vi "Measurements Graph_Seperated Ports.vi"(0 "Resitance":dbl[](array[numeric])=[0.1, 0.1, 0.3, 0.28, 0.18, 0.08], 1 "Bias Voltage":dbl[](array[numeric])=[0.0, 1.0, 2.0, 2.0, 1.0, 0.0], 2 "Stop_V":dbl, 5 "P1":dbl[](array[numeric])=[10.0, 11.0, 12.0, 11.75, 10.85, 9.5], 7 "P2":dbl[](array[numeric])=[20.0, 21.0, 22.0, 21.75, 20.35, 18.65], 9 "P3":dbl[](array[numeric])=[30.0, 31.0, 32.0, 31.5, 30.47, 29.42], 11 "Error In":errorcluster) -> (4 "Graph Cluster":T1, 15 "Error Out":errorcluster)   [LabVIEW 2013]
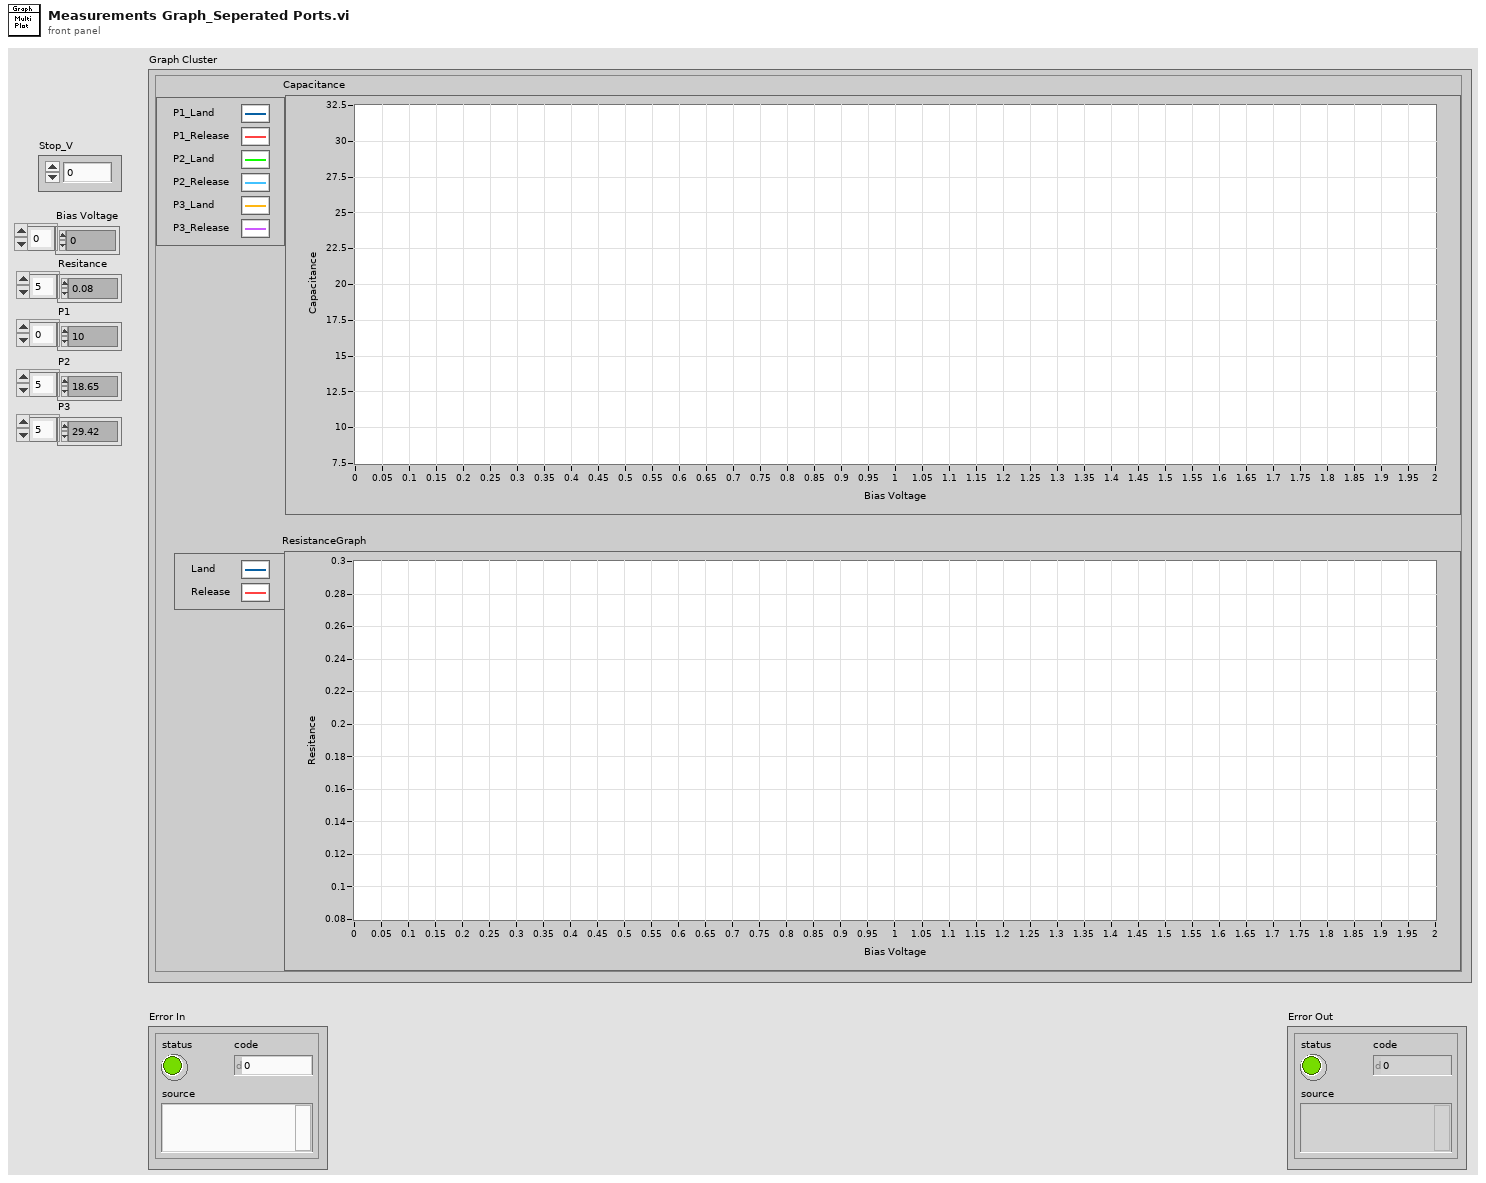
[diagram p1: front panel]
types:
  T1 = cluster{"ResistanceGraph":cluster{dbl[], dbl[]}[], "Capacitance":cluster{dbl[], dbl[]}[]}
  T2 = cluster{cluster{dbl[], dbl[]}[], cluster{dbl[], dbl[]}[]}
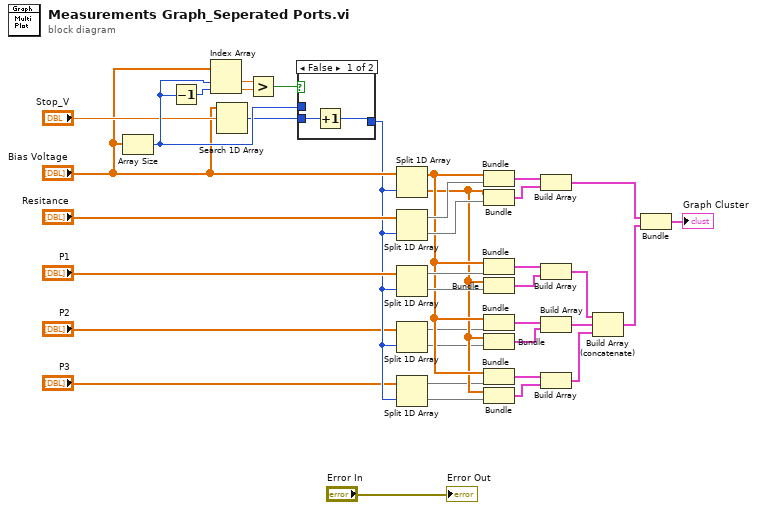
[diagram p0: block diagram]
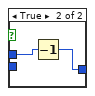
[diagram p2: hidden frame]
diagram:
  n1 = Array Size(array="Bias Voltage") -> (size(s)=w24:i32)
  n2 = Decrement(x=w24) -> (x-1=w27:i32)
  n3 = Index Array(array="Bias Voltage", index #1=w24, index #2=w27) -> (element #1=w25:dbl, element #2=w26:dbl)
  n4 = Search 1D Array(1D array="Bias Voltage", element="Stop_V") -> (index of element=w21:i32)  [unwired: 1 in]
  n5 = Greater?(x=w25, y=w26) -> (0:w20:bool)
  n6 = case shown="False" w20 {
    tunnel: w24 -> [_ w42]
    tunnel: [w39 w41] -> w17
    tunnel: w21 -> [w40 _]
    frame False {
      n7 = Increment(x=w40) -> (x+1=w39:i32)
    }
    frame True {
      n8 = Decrement(x=w42) -> (x-1=w41:i32)
    }
  }
  n9 = Split 1D Array(array="Bias Voltage", index=w17) -> (first subarray=w15:dbl[], second subarray=w14:dbl[])
  n10 = Split 1D Array(array="Resitance", index=w17) -> (first subarray=w37:dbl[], second subarray=w36:dbl[])
  n11 = Split 1D Array(array="P1", index=w17) -> (first subarray=w31:dbl[], second subarray=w30:dbl[])
  n12 = Split 1D Array(array="P2", index=w17) -> (first subarray=w13:dbl[], second subarray=w12:dbl[])
  n13 = Split 1D Array(array="P3", index=w17) -> (first subarray=w11:dbl[], second subarray=w10:dbl[])
  n14 = Bundle(w15, w37) -> (w35:cluster{dbl[], dbl[]})  [unwired: 1 in]
  n15 = Bundle(w14, w36) -> (w34:cluster{dbl[], dbl[]})  [unwired: 1 in]
  n16 = Bundle(w15, w31) -> (w33:cluster{dbl[], dbl[]})  [unwired: 1 in]
  n17 = Bundle(w14, w30) -> (w32:cluster{dbl[], dbl[]})  [unwired: 1 in]
  n18 = Bundle(w15, w13) -> (w8:cluster{dbl[], dbl[]})  [unwired: 1 in]
  n19 = Bundle(w14, w12) -> (w7:cluster{dbl[], dbl[]})  [unwired: 1 in]
  n20 = Bundle(w15, w11) -> (w6:cluster{dbl[], dbl[]})  [unwired: 1 in]
  n21 = Bundle(w14, w10) -> (w5:cluster{dbl[], dbl[]})  [unwired: 1 in]
  n22 = Build Array(w35, w34) -> (w29:cluster{dbl[], dbl[]}[])
  n23 = Build Array(w33, w32) -> (w4:cluster{dbl[], dbl[]}[])
  n24 = Build Array(w8, w7) -> (w3:cluster{dbl[], dbl[]}[])
  n25 = Build Array(w6, w5) -> (w2:cluster{dbl[], dbl[]}[])
  n26 = Build Array (concatenate)(w4, w3, w2) -> (w1:cluster{dbl[], dbl[]}[])
  n27 = Bundle(w29, w1) -> (→"Graph Cluster":T2)  [unwired: 1 in]
  "Error Out" <- "Error In"
